vi "proiectu fara drona.vi"() -> ()   [LabVIEW 2015]
uses:
  BmpWork/lee_4/bin/Debug/lee_4.dll
  LEE/lee_30_10_2016/bin/Debug/lee_30_10_2016.dll
panel:
  in  "Numeric":u32
  out "Curently at image:":string
  out "Started creating image from matrix":bool
  in  "START":bool
  out "Image 2":T1(plugin-control)
  out "Image":T1(plugin-control)
  out "Computing Path for the car":bool
  out "Finding START/STOP":bool
  out "Started stitching":bool
  out "Started normalising and cropping":bool
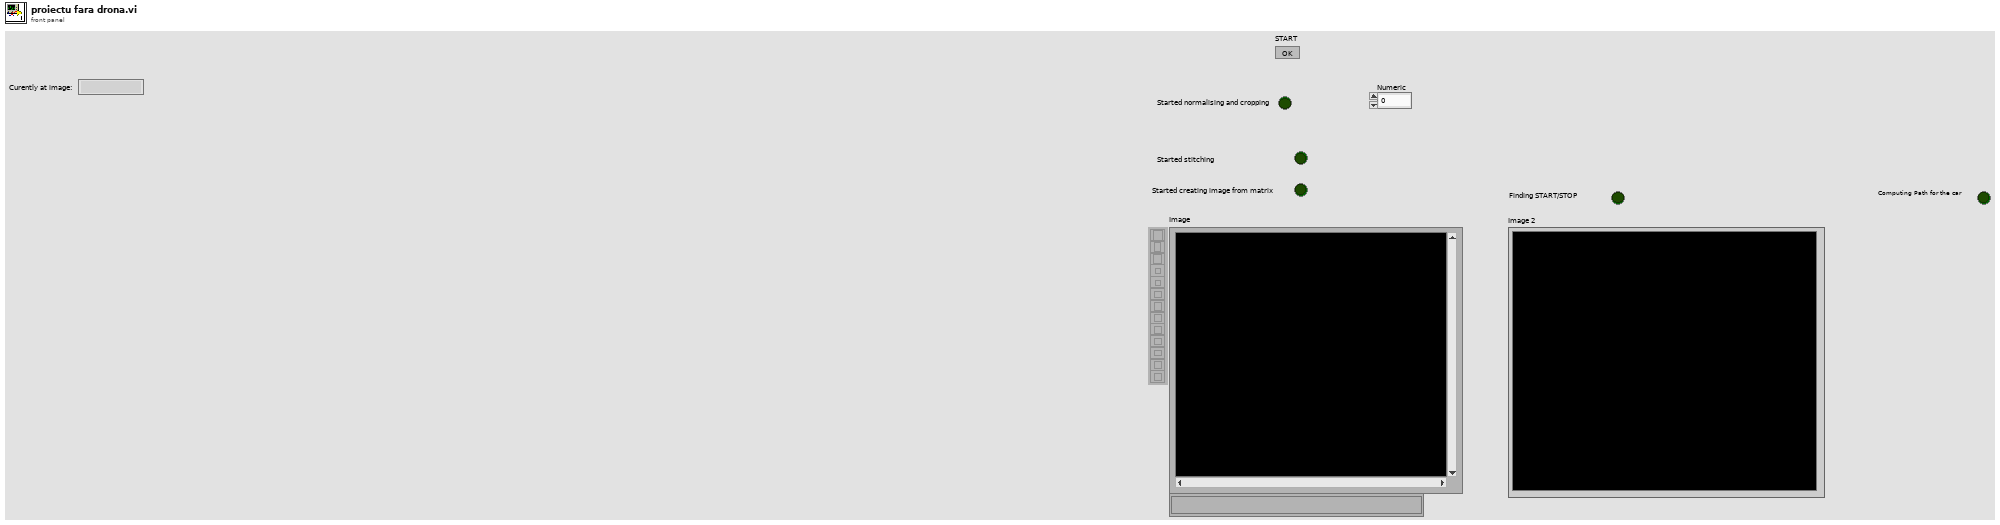
[diagram p1: front panel]
types:
  T1 = typedef "IMAQ Image.ctl" = refnum<image>
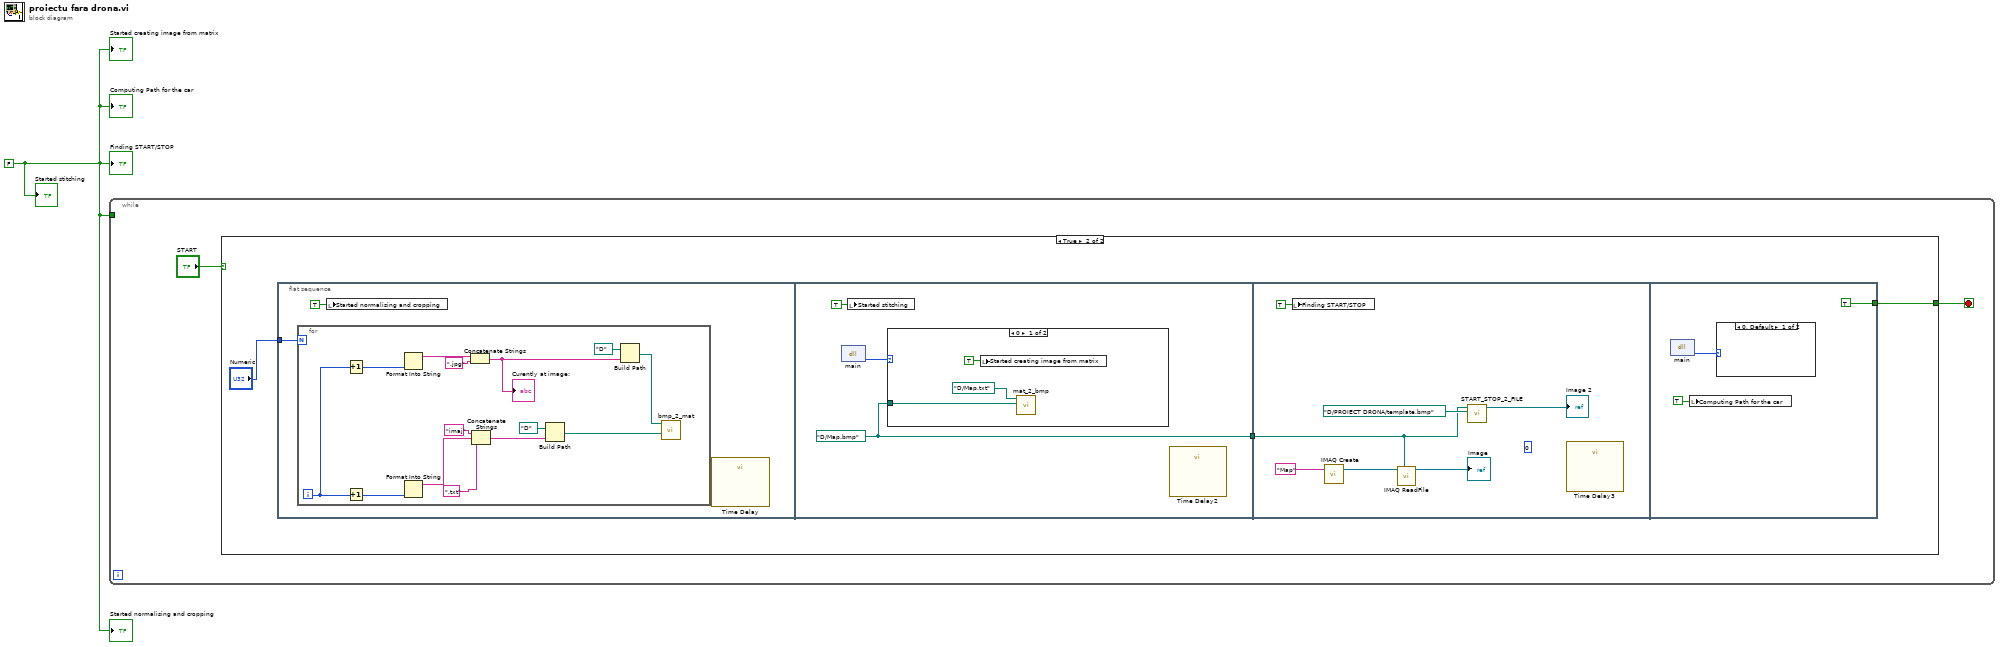
[diagram p0: block diagram]
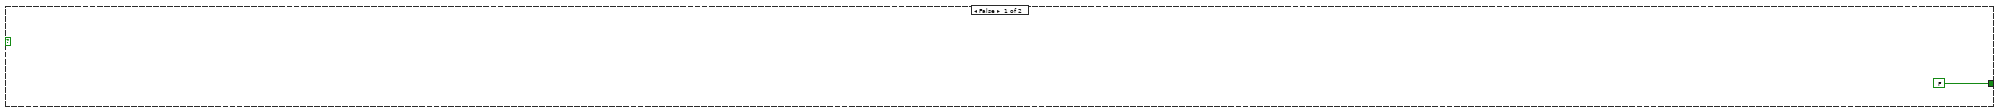
[diagram p2: hidden frame]
diagram:
  w1 = FALSE
  n1 = while {
    tunnel: w1 -> [_]
    stop <- w2 stop-if-true
    n2 = case shown="True" "START" {
      tunnel: [FALSE w6] -> w2
      frame False {
      }
      frame True {
        n3 = flat-sequence {
          tunnel: "Numeric" -> [w8]
          tunnel: [w25] -> w7
          tunnel: w7 -> [w33]
          tunnel: [TRUE] -> w6
          frame #0 {
            n4 = for {
              N: w8 -> [_]
              i -> [w10]
              n5 = Increment(x=w10) -> (x+1=w14:i32)
              n6 = Increment(x=w10) -> (x+1=w13:i32)
              n7 = Format Into String(w14) -> (resulting string=w22:string)  [unwired: 3 in, 1 out]
              n8 = Format Into String(w13) -> (resulting string=w19:string)  [unwired: 3 in, 1 out]
              n9 = Concatenate Strings(w22, ".jpg" ("string")) -> (w11:string)
              "Curently at image:" <- w11
              n10 = Concatenate Strings("imaj" ("string"), w19, ".txt" ("string")) -> (w16:string)
              n11 = Build Path(base path=path "D:/", name or relative path=w16) -> (appended path=w15:path)
              n12 = Build Path(base path=path "D:/", name or relative path=w11) -> (appended path=w12:path)
              n13 = call "bmp_2_mat.vi"("Destinatia1"=w15, "Imaginea1"=w12) -> ()  [unwired: 10 in]
            }
            n14 = local write "Started normalising and cropping"(TRUE) -> ()
            n15 = call "Time Delay"() -> ()  [unwired: 11 in, 1 out]
          }
          frame #1 {
            w25 = path "D:/Map.bmp" ("Fisierul Text")
            n16 = dll-call lib="D:/PROIECT DRONA/BmpWork/lee_4/bin/Debug/lee_4.dll" fn="main"() -> ("return type"=w26:i32)  [unwired: 3 in, 2 out]
            n17 = local write "Started stitching"(TRUE) -> ()
            n18 = case shown="0" w26 {
              tunnel: w25 -> [w29 _]
              frame 0 {
                n19 = local write "Started creating image from matrix"(TRUE) -> ()
                n20 = call "mat_2_bmp.vi"("Path"=w29, "Path 7"=path "D:/Map.txt" ("Fisierul Text")) -> ()  [unwired: 10 in]
              }
              frame 2, Default {
              }
            }
            n21 = call "Time Delay2"() -> ()  [unwired: 11 in, 1 out]
          }
          frame #2 {
            (unwired) 0 ("index")
            n22 = local write "Finding START/STOP"(TRUE) -> ()
            n23 = call "IMAQ Create"("Image Name"="Map") -> ("New Image"=w32:T1)  [unwired: 4 in, 1 out]
            n24 = call "IMAQ ReadFile"("File Path"=w33, "Image"=w32) -> ("Image Out"=→"Image":T1)  [unwired: 5 in, 4 out]
            n25 = call "START_STOP_2_FILE.vi"("Template"=path "D:/PROIECT DRONA/template.bmp" ("Path to template"), "MAP"=w33) -> ("Image"=→"Image 2":T1)  [unwired: 9 in]
            n26 = call "Time Delay3"() -> ()  [unwired: 11 in, 1 out]
          }
          frame #3 {
            n27 = dll-call lib="D:/PROIECT DRONA/LEE/lee_30_10_2016/bin/Debug/lee_30_10_2016.dll" fn="main"() -> ("return type"=w39:i32)  [unwired: 3 in, 2 out]
            n28 = local write "Computing Path for the car"(TRUE) -> ()
            n29 = case shown="0, Default" w39 {
              frame 0, Default {
              }
              frame 4 {
              }
            }
          }
        }
      }
    }
  }
  "Finding START/STOP" <- w1
  "Computing Path for the car" <- w1
  "Started stitching" <- w1
  "Started normalising and cropping" <- w1
  "Started creating image from matrix" <- w1
